vi "Demo - Read AI Channel 0.vi"() -> ()   [LabVIEW 2020]
uses:
  TypeDefs/Enum - Machine State.ctl
  <vilib>/ErrorRing/Error Ring.xnode
panel:
  out "Program Status":string
  in  "Stop":bool
  out "Waveform Chart":dbl(graph)
  in  "DAQ IP Address":string="192.168.1.1"
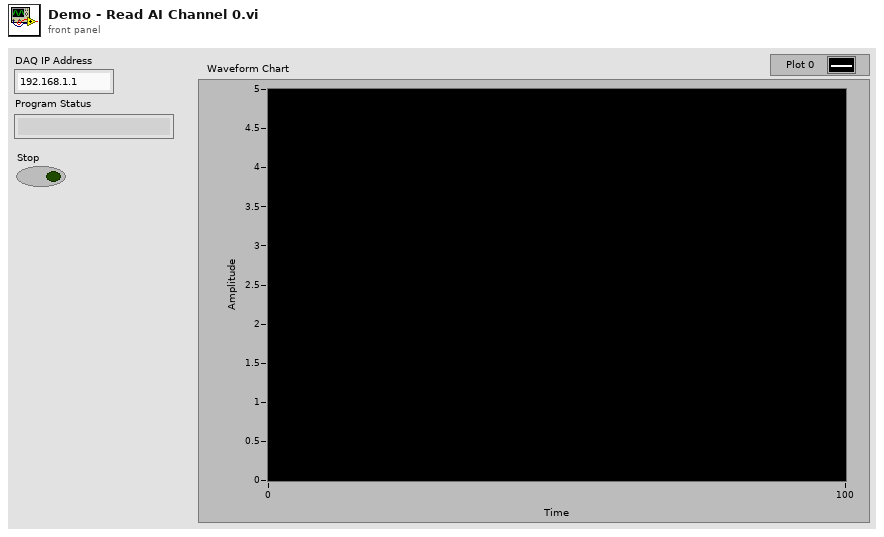
[diagram p1: front panel]
types:
  T1 = typedef "Enum - Machine State.ctl" = enum16{"Shutdown", "Start Streaming", "Initialize", "Read Streamed Data"}
  T2 = typedef "TypeDef - Cluster Representing Decoded JSON Message.ctl" = cluster{"timestamp":u64, "adc":cluster{"time":i32, "ch":i32, "data":i32}[], "dio":cluster{"time":i32, "mask":i32, "data":u16}[]}
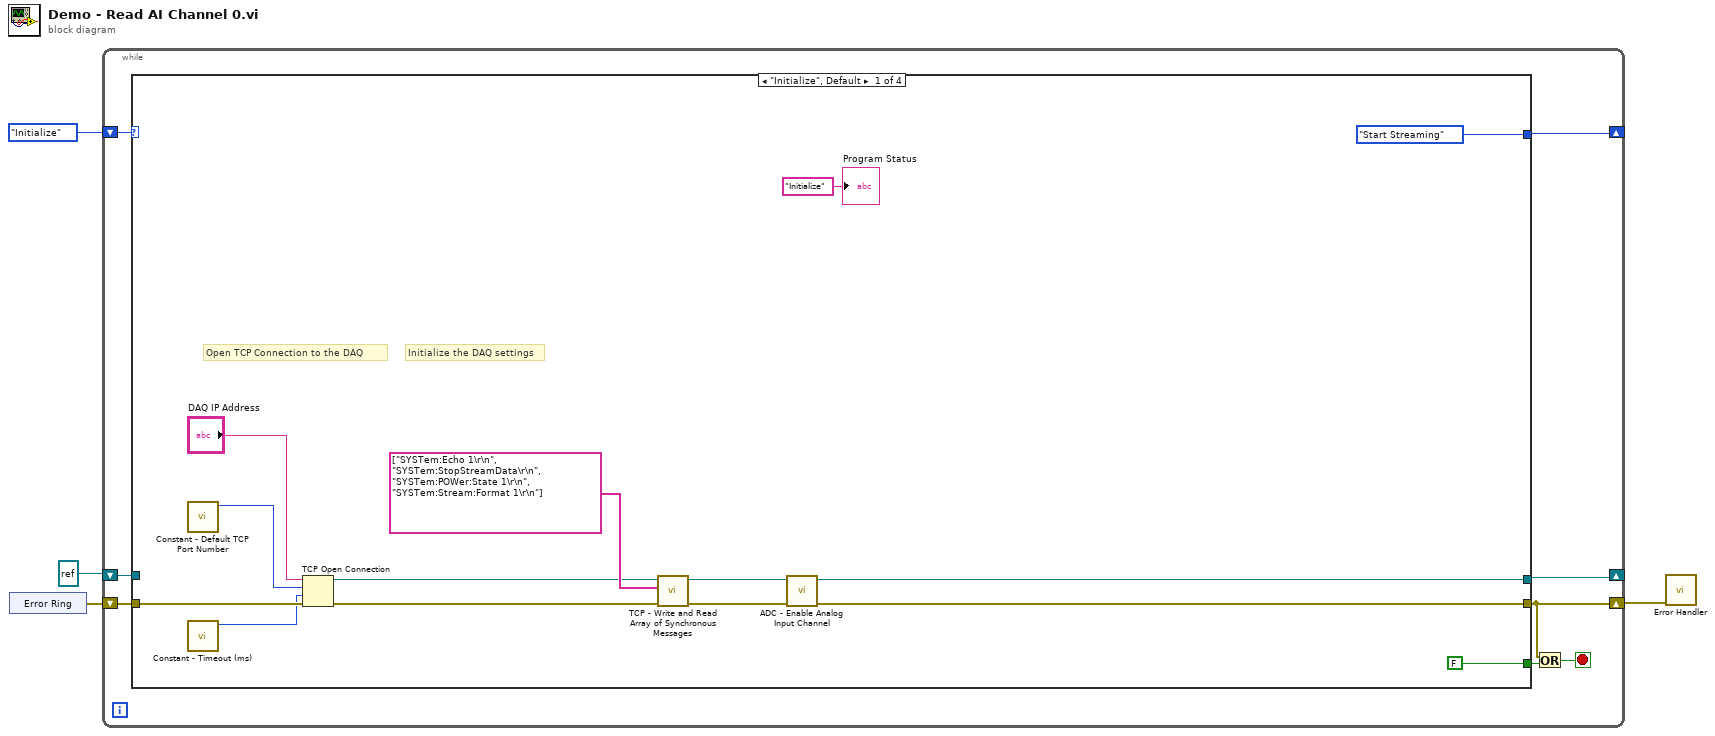
[diagram p0: block diagram]
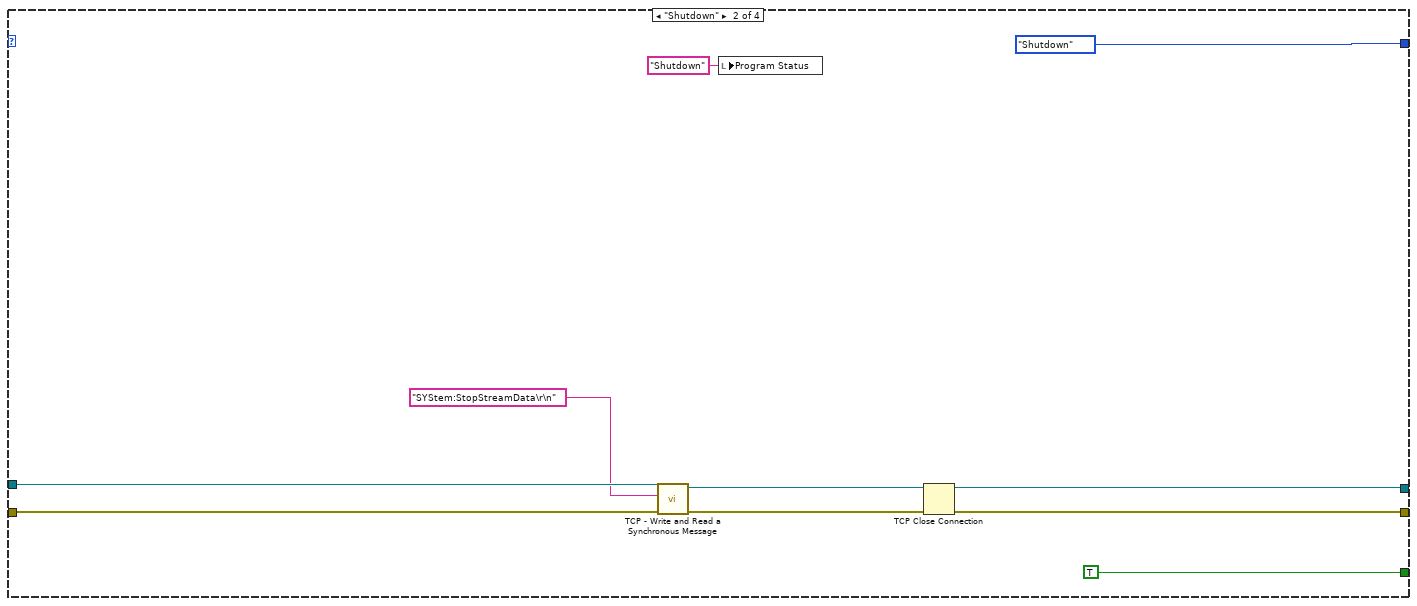
[diagram p2: hidden frame]
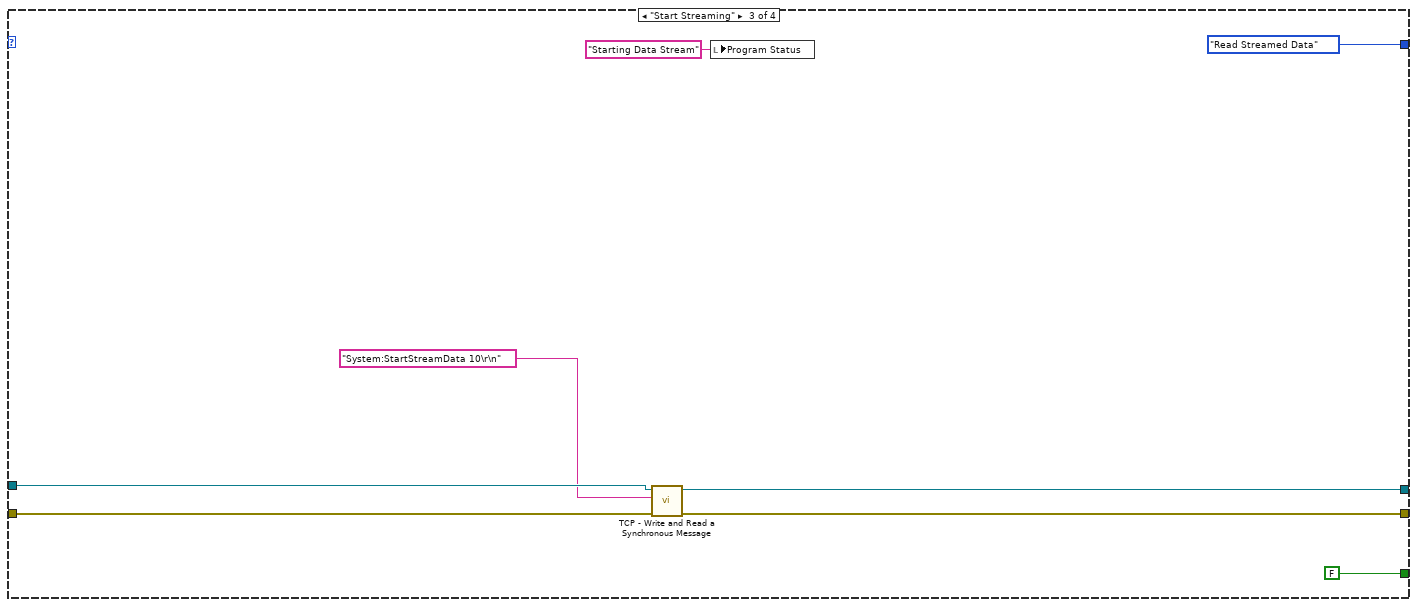
[diagram p3: hidden frame]
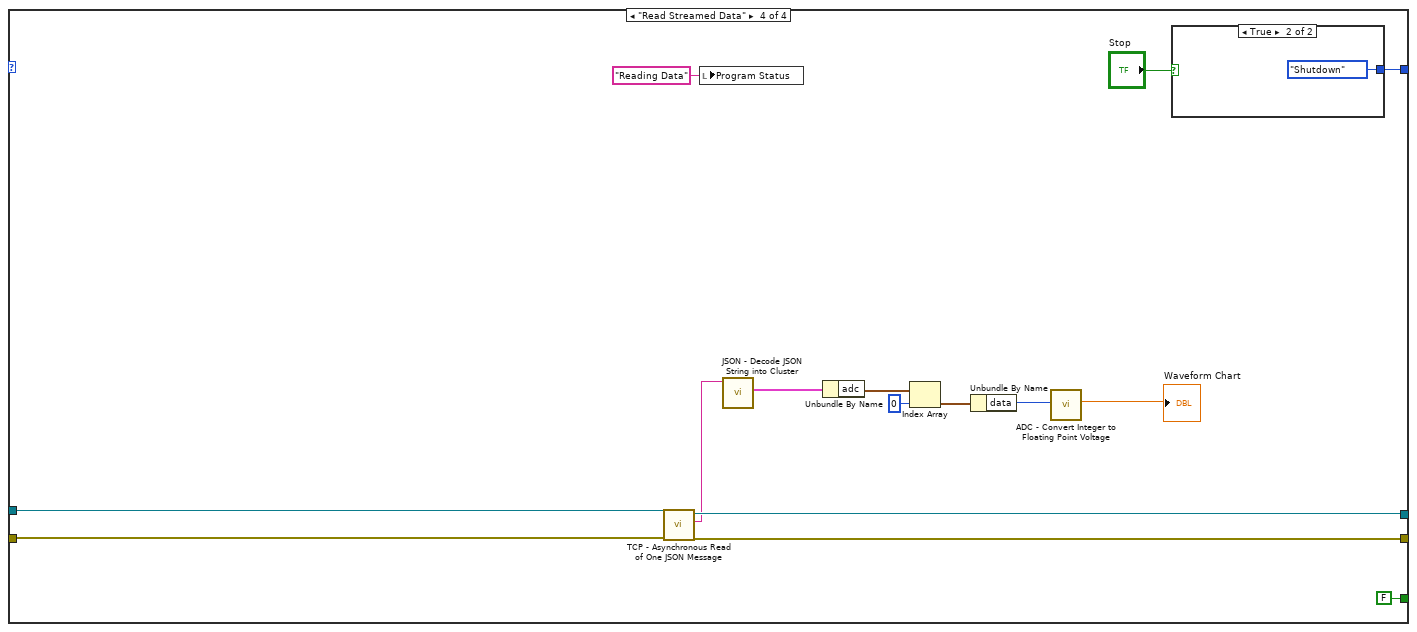
[diagram p4: hidden frame]
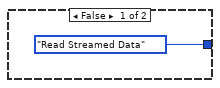
[diagram p5: hidden frame]
diagram:
  n1 = xnode "Error Ring"() -> ("error out"=w3:errorcluster)
  n2 = while {
    shift-right: [w6] -> w1
    shift-left: w3 -> [w11]
    shift-right: [w10] -> _
    shift-left: refnum<k5> refnum ("TCP Network Connection out") -> [w8]
    shift-right: [w9] -> _
    shift-left: Enum_-_Machine_State."Initialize" -> [w12]
    stop <- w5 stop-if-true
    n3 = case shown="\"Initialize\", Default" w12 {
      tunnel: w11 -> [w24 w33 w44 w55]
      tunnel: [w14 w28 w43 w56] -> w6
      tunnel: [w15 w29 w42 w57] -> w10
      tunnel: [Enum_-_Machine_State."Start Streaming" Enum_-_Machine_State."Shutdown" Enum_-_Machine_State."Read Streamed Data" w59] -> w9
      tunnel: [FALSE TRUE FALSE FALSE] -> w7
      tunnel: w8 -> [_ w34 w41 w58]
      frame "Initialize", Default {
        # "Open TCP Connection to the DAQ"
        # "Initialize the DAQ settings"
        n4 = call "Constant - Default TCP Port Number.vi"() -> ("Port"=w25:u16)  [unwired: 11 in]
        n5 = call "Constant - Timeout (ms).vi"() -> ("timeout (ms)"=w16:i32)  [unwired: 11 in]
        n6 = TCP Open Connection(address="DAQ IP Address", remote port or service name=w25, timeout ms (60000)=w16, error in (no error)=w24) -> (connection ID=w21:refnum<k5>, error out=w22:errorcluster)  [unwired: 1 in]
        n7 = call "TCP - Write and Read Array of Synchronous Messages.vi"("error in"=w22, "Array of Messages to Send"=string[] ["SYSTem:Echo 1\r\n", "SYSTem:StopStreamData\r\n", "SYSTem:POWer:State 1\r\n", "SYSTem:Stream:Format 1\r\n"], "TCP Network Connection in"=w21) -> ("error out"=w17:errorcluster, "TCP Network Connection out"=w18:refnum<k5>)  [unwired: 6 in, 1 out]
        n8 = call "ADC - Enable Analog Input Channel.vi"("error in (no error)"=w17, "TCP Network Connection in"=w18) -> ("error out"=w14:errorcluster, "TCP Network Connection out"=w15:refnum<k5>)  [unwired: 8 in]
        "Program Status" <- "Initialize" ("Program Status")
      }
      frame "Shutdown" {
        n9 = call "TCP - Write and Read a Synchronous Message.vi"("error in"=w33, "Message to Send"="SYStem:StopStreamData\r\n", "TCP Network Connection in"=w34) -> ("error out"=w30:errorcluster, "TCP Network Connection out"=w31:refnum<k5>)  [unwired: 6 in, 1 out]
        n10 = local write "Program Status"("Shutdown" ("Program Status")) -> ()
        n11 = TCP Close Connection(connection ID=w31, error in (no error)=w30) -> (connection ID out=w29:refnum<k5>, error out=w28:errorcluster)  [unwired: 1 in]
      }
      frame "Start Streaming" {
        n12 = call "TCP - Write and Read a Synchronous Message.vi"("error in"=w44, "Message to Send"="System:StartStreamData 10\r\n" ("data in"), "TCP Network Connection in"=w41) -> ("error out"=w43:errorcluster, "TCP Network Connection out"=w42:refnum<k5>)  [unwired: 6 in, 1 out]
        n13 = local write "Program Status"("Starting Data Stream" ("Program Status")) -> ()
      }
      frame "Read Streamed Data" {
        n14 = call "TCP - Asynchronous Read of One JSON Message.vi"("error in"=w55, "TCP Network Connection in"=w58) -> ("error out"=w56:errorcluster, "Received JSON Message"=w54:string, "TCP Network Connection out"=w57:refnum<k5>)  [unwired: 7 in]
        n15 = local write "Program Status"("Reading Data" ("Program Status")) -> ()
        n16 = call "JSON - Decode JSON String into Cluster.vi"("JSON String"=w54) -> ("Data out"=w53:T2)  [unwired: 9 in, 1 out]
        n17 = Unbundle By Name(w53) -> ("adc"=w52:cluster{"time":i32, "ch":i32, "data":i32}[])
        n18 = Index Array(array=w52, index=0) -> (element=w50:cluster{"time":i32, "ch":i32, "data":i32})
        n19 = Unbundle By Name(w50) -> ("data"=w47:i32)
        n20 = call "ADC - Convert Integer to Floating Point Voltage.vi"("Analog Integer Value In"=w47) -> ("Analog Voltage (V)"=→"Waveform Chart":dbl)  [unwired: 10 in]
        n21 = case shown="True" "Stop" {
          tunnel: [Enum_-_Machine_State."Read Streamed Data" Enum_-_Machine_State."Shutdown"] -> w59
          frame False {
          }
          frame True {
          }
        }
      }
    }
    n22 = Or(x=w6, y=w7) -> (x .or. y?=w5:bool)
  }
  n23 = call "Error Handler.vi"("error in"=w1) -> ()  [unwired: 10 in, 1 out]
